vi "add.vi"(11 "LabVIEW Web Service Request":refnum<class "Web Request.lvclass">) -> (3 "sum":dbl)   [LabVIEW 2014]
uses:
  <vilib>/wsapi/Web Request.lvclass
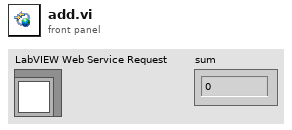
[diagram p1: front panel]
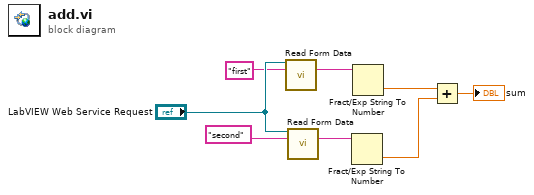
[diagram p0: block diagram]
diagram:
  n1 = call <vilib>:"Read Form Data.vi"("LabVIEW Web Service Request"="LabVIEW Web Service Request", "key"="first") -> ("value"=w3:string)  [unwired: 10 in, 3 out]
  n2 = call <vilib>:"Read Form Data.vi"("LabVIEW Web Service Request"="LabVIEW Web Service Request", "key"="second") -> ("value"=w4:string)  [unwired: 10 in, 3 out]
  n3 = Fract/Exp String To Number(string=w4) -> (number=w1:dbl)  [unwired: 3 in, 1 out]
  n4 = Fract/Exp String To Number(string=w3) -> (number=w2:dbl)  [unwired: 3 in, 1 out]
  n5 = Add(x=w2, y=w1) -> (x+y=→"sum":dbl)
